vi "Ex6_Serrure_Num_2_MDP.vi"() -> ()   [LabVIEW 2018]
panel:
  out "Numeric":dbl
  in  "String":string
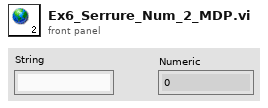
[diagram p1: front panel]
diagram:
